vi "verify unique value in a list.vi"(7 "parameter name":string, 8 "error in (no error)":errorcluster, 9 "value":u16, 10 "list of values":u16[](array[numeric]), 11 "Simulated_CCD_Camera in":refnum<class "Simulated Camera.lvclass">) -> (0 "error out":errorcluster, 3 "Simulated_CCD_Camera out":refnum<class "Simulated Camera.lvclass">)   [LabVIEW 2018, in "Simulated Camera.lvclass"]
uses:
  Simulated Camera.lvclass
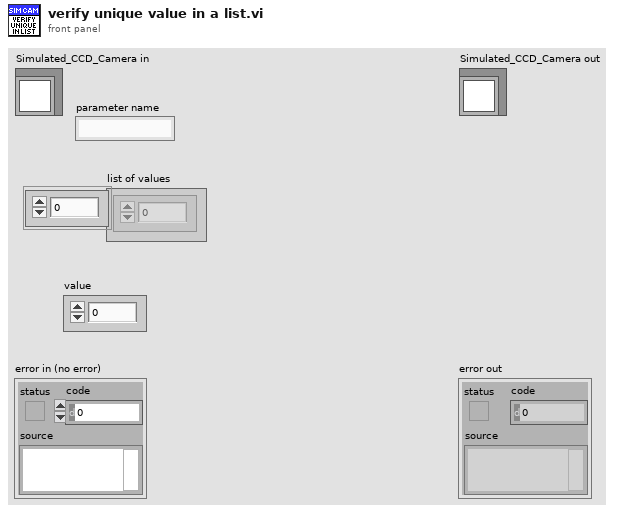
[diagram p1: front panel]
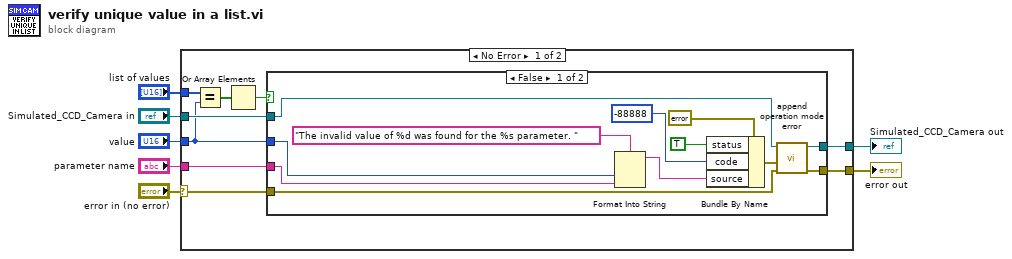
[diagram p0: block diagram]
diagram:
  n1 = case shown="No Error" "error in (no error)" {
    selector: "error in (no error)" -> [w9 w32]
    tunnel: [w8 w32] -> w6
    tunnel: [w12 w31] -> w4
    tunnel: "Simulated_CCD_Camera in" -> [w13 w31]
    tunnel: "list of values" -> [w16 _]
    tunnel: "value" -> [w10 _]
    tunnel: "parameter name" -> [w11 _]
    frame No Error {
      n2 = Equal?(x=w16, y=w10) -> (x = y?=w15:bool[])
      n3 = Or Array Elements(Boolean array=w15) -> (logical OR=w14:bool)
      n4 = case shown="False" w14 {
        tunnel: w13 -> [w20 w30]
        tunnel: [w21 w30] -> w12
        tunnel: w11 -> [w24 _]
        tunnel: w10 -> [w22 _]
        tunnel: w9 -> [w19 w29]
        tunnel: [w18 w29] -> w8
        frame False {
          n5 = Format Into String(format string="The invalid value of %d was found for the %s parameter. " ("source"), w22, w24) -> (resulting string=w23:string)  [unwired: 2 in, 1 out]
          n6 = Bundle By Name(cluster=errorcluster {"status"=FALSE, "code"=0, "source"=""} ("error constant"), "status"=TRUE, "code"=-88888, "source"=w23) -> (w17:errorcluster)
          n7 = call "append operation mode error.vi"("error in (no error)"=w19, "error"=w17, "Simulated_CCD_Camera in"=w20) -> ("error out"=w18:errorcluster, "Simulated_CCD_Camera out"=w21:refnum<class "Simulated Camera.lvclass">)  [unwired: 7 in]
        }
        frame True {
        }
      }
    }
    frame Error {
    }
  }
  "error out" <- w6
  "Simulated_CCD_Camera out" <- w4
